vi "Create (Replace) File.vi"(8 "error in":errorcluster, 10 "Path":path, 11 "File Session in":refnum<class "File Session.lvclass">) -> (0 "error out":errorcluster, 3 "File Session out":refnum<class "File Session.lvclass">)   [LabVIEW 2015, in "File Session.lvclass"]
doc: "Opens a reference to a file by creating or replacing the file defined by path. If the directory for which the file is intended does not exist, then that directory will be created."
uses:
  File Session.lvclass
  File Session.lvclass/File Session.ctl
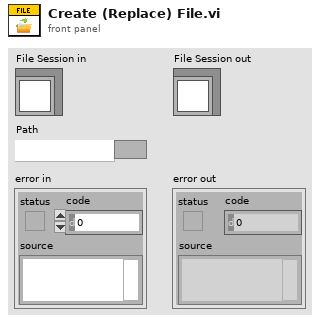
[diagram p1: front panel]
types:
  T1 = enum16{"open", "replace", "create", "open or create", "replace or create", "replace or create with confirmation"}
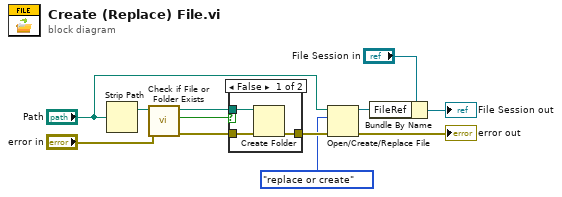
[diagram p0: block diagram]
diagram:
  n1 = Strip Path(path="Path") -> (stripped path=w12:path)  [unwired: 1 out]
  n2 = call <vilib>:"Check if File or Folder Exists.vi"("error in (no error)"="error in", "path"=w12) -> ("error out"=w8:errorcluster, "file or folder exists?"=w11:bool, "dup path"=w9:path)  [unwired: 7 in]
  n3 = case shown="False" w11 {
    tunnel: w9 -> [w15 _]
    tunnel: w8 -> [w14 w16]
    tunnel: [w13 w16] -> w6
    frame False {
      n4 = Create Folder(path (use dialog)=w15, error in=w14) -> (error out=w13:errorcluster)  [unwired: 1 in, 2 out]
    }
    frame True {
    }
  }
  n5 = Open/Create/Replace File(file path (use dialog)="Path", error in=w6, operation (0:open)=T1."replace or create") -> (refnum out=w2:refnum<file>, error out=→"error out":errorcluster)  [unwired: 3 in, 1 out]
  n6 = Bundle By Name(cluster="File Session in", "FileRef"=w2) -> (→"File Session out":refnum<class "File Session.lvclass">)
